vi "NO ZERO VALUES(SubVI).vi"(1 "Numeric":dbl) -> (0 "t":dbl)   [LabVIEW 2019]
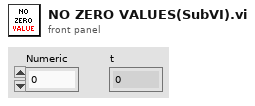
[diagram p1: front panel]
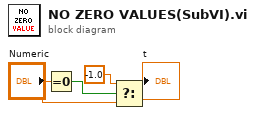
[diagram p0: block diagram]
diagram:
  n1 = Equal To 0?(x="Numeric") -> (x = 0?=w1:bool)
  n2 = Select(t=-1.0, s=w1, f="Numeric") -> (s? t:f=→"t":dbl)
